vi "__AttSet_11713A.vi"(0 "ATT(dB)":i16=79, 3 "GPIB":string="28") -> ()   [LabVIEW 2017]
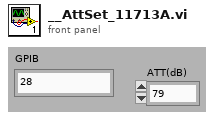
[diagram p1: front panel]
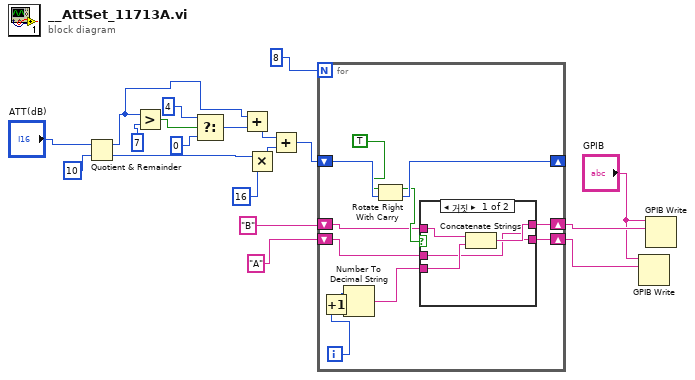
[diagram p0: block diagram]
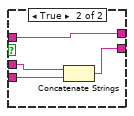
[diagram p2: hidden frame]
diagram:
  n1 = Quotient & Remainder(x="ATT(dB)", y=10) -> (x-y*floor(x/y)=w1:i32, floor(x/y)=w17:i32)
  n2 = Greater?(x=w1, y=7) -> (0:w6:bool)
  n3 = Select(t=4, s=w6, f=0) -> (s? t:f=w3:i32)
  n4 = Add(x=w1, y=w3) -> (x+y=w2:i32)
  n5 = Multiply(x=w17, y=16) -> (x*y=w11:i32)
  n6 = Add(x=w2, y=w11) -> (x+y=w12:i32)
  n7 = for {
    N: 8 -> [_]
    shift-right: [w29] -> _
    shift-left: w12 -> [w30]
    shift-right: [w24] -> w8
    shift-left: "A" -> [w26]
    shift-right: [w23] -> w10
    shift-left: "B" -> [w22]
    i -> [w27]
    n8 = Increment(x=w27) -> (x+1=w20:i32)
    n9 = Number To Decimal String(number=w20) -> (decimal integer string=w25:string)  [unwired: 1 in]
    n10 = Rotate Right With Carry(2:w30, 3:TRUE) -> (0:w29:i32, 1:w28:bool)
    n11 = case shown="거짓" w28 {
      tunnel: w26 -> [w31 w38]
      tunnel: w25 -> [w32 w37]
      tunnel: [w31 w36] -> w24
      tunnel: [w33 w35] -> w23
      tunnel: w22 -> [w34 w35]
      frame False {
        n12 = Concatenate Strings(w34, w32) -> (w33:string)
      }
      frame True {
        n13 = Concatenate Strings(w38, w37) -> (w36:string)
      }
    }
  }
  n14 = GPIB Write(0:"GPIB", 1:w8) -> ()  [unwired: 3 in, 2 out]
  n15 = GPIB Write(0:"GPIB", 1:w10) -> ()  [unwired: 3 in, 2 out]
